vi "MathCad cmd v2.vi"(4 "Arr Refnum":refnum<vi>, 5 "MathCAD variables":T1, 6 "MathCAD cmds":T2, 7 "Str Refnum":refnum<vi>, 8 "error in":errorcluster, 9 "Clust Refnum":refnum<vi>, 10 "Num Refnum":refnum<vi>) -> (0 "first error out":errorcluster, 1 "errors":errorcluster[](array[cluster]))   [LabVIEW 2011, in "Design Server.lvlib"]
uses:
  Design Server.lvlib
  MathCAD cmd.ctl
  MathCAD results ref.ctl
panel:
  in  "Worksheet":path=path "C:/Users/design/Documents/Final Designs/AguaClaraDesignTool.xmcd"
  in  "Mathcad.IMathcadApplication":refnum<k7>
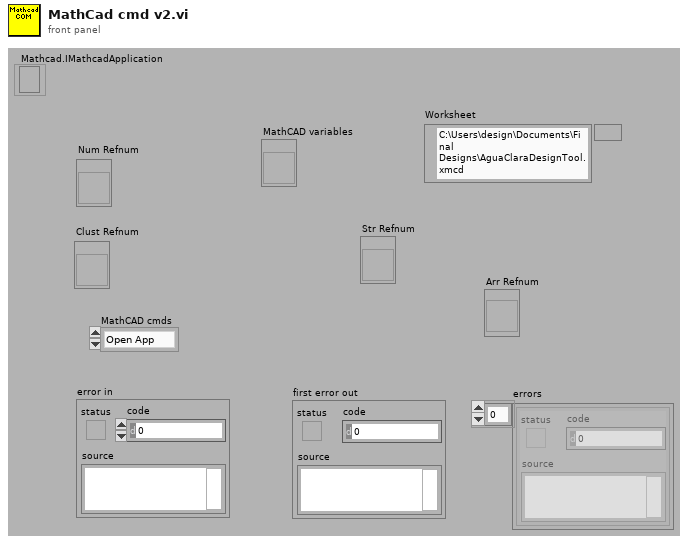
[diagram p1: front panel]
types:
  T1 = typedef "Design Server.lvlib/MathCAD results ref.ctl" = refnum<vi>
  T2 = typedef "Design Server.lvlib/MathCAD cmd.ctl" = enum16{"Open App", "Open Worksheet", "Close Worksheet", "Load Variable Ref", "Send Number", "Send Cluster", "Send Array", "Send String", "Calculate", "Get MathCAD data", "Close MathCAD"}
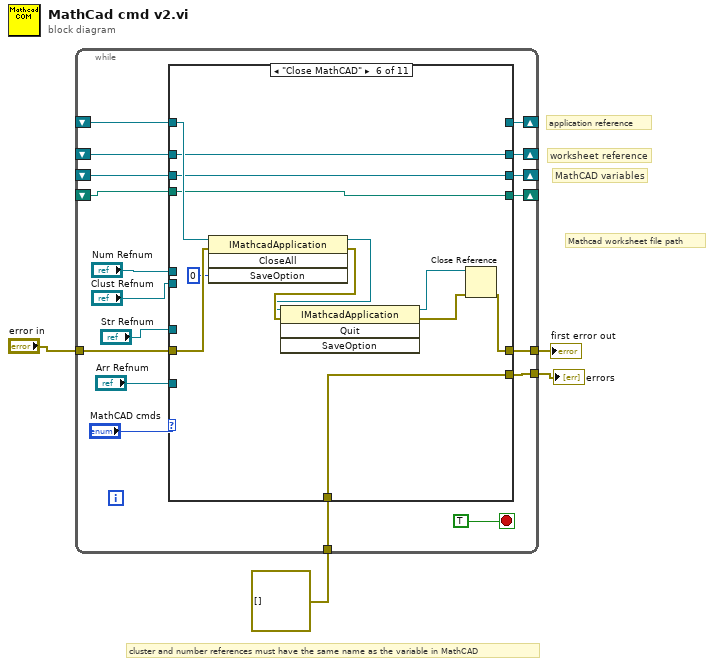
[diagram p0: block diagram]
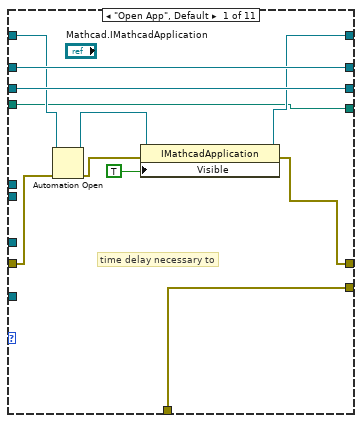
[diagram p2: hidden frame]
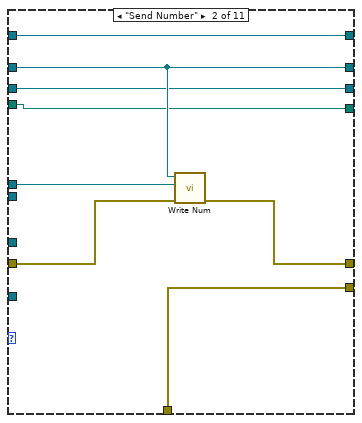
[diagram p3: hidden frame]
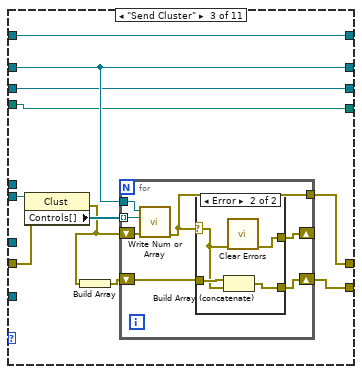
[diagram p4: hidden frame]
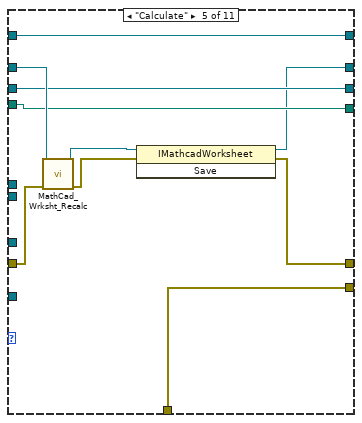
[diagram p7: hidden frame]
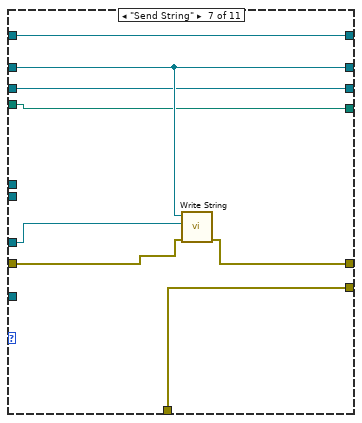
[diagram p8: hidden frame]
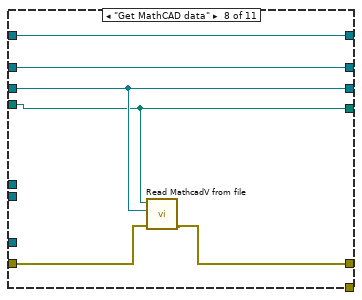
[diagram p9: hidden frame]
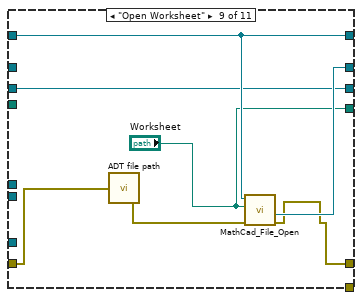
[diagram p10: hidden frame]
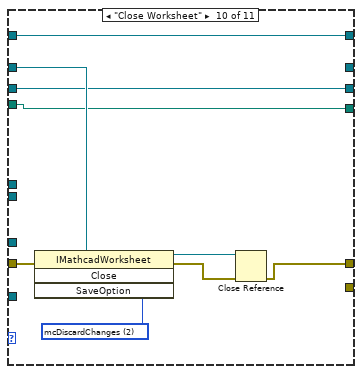
[diagram p11: hidden frame]
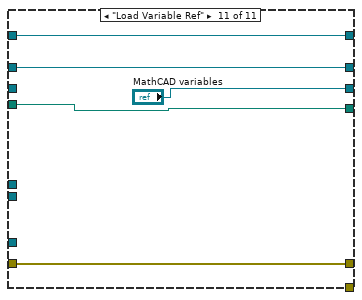
[diagram p12: hidden frame]
diagram:
  # "Mathcad worksheet file path"
  # "MathCAD variables"
  # "application reference"
  # "worksheet reference"
  # "cluster and number references must have the same name as the variable in MathCAD"
  n1 = while {
    shift-right: [w18] -> _
    shift-left: _ -> [w16]
    shift-right: [w17] -> _
    shift-left: _ -> [w15]
    tunnel: "error in" -> [w19]
    tunnel: [w20] -> w3
    tunnel: [w10] -> w2
    tunnel: errorcluster[] [] -> [w9]
    shift-right: [w8] -> _
    shift-left: _ -> [w7]
    shift-right: [w6] -> _
    shift-left: _ -> [w5]
    stop <- TRUE stop-if-true
    n2 = case shown="\"Close MathCAD\"" "MathCAD cmds" {
      tunnel: [w26 w38 w49 w69 w72 w88 w99 w104 w109 w116 w125] -> w20
      tunnel: w19 -> [w25 w40 w47 w69 w79 w92 w100 w105 w112 w123 w125]
      tunnel: [w27 w41 w51 w71 w81 _ w101 w107 w114 w120 w126] -> w18
      tunnel: [w32 w39 w50 w70 w74 w91 w97 w106 w113 _ w127] -> w17
      tunnel: w16 -> [w30 w41 w51 w71 w81 w93 w101 w107 w114 w120 w126]
      tunnel: w15 -> [w32 w39 w50 w70 w80 w91 w97 w106 _ w121 w127]
      tunnel: "Num Refnum" -> [_ w37 _ _ _ _ _ _ _ _ _]
      tunnel: "Clust Refnum" -> [_ _ w48 _ _ _ _ _ _ _ _]
      tunnel: "Str Refnum" -> [_ _ _ _ _ _ w98 _ _ _ _]
      tunnel: "Arr Refnum" -> [_ _ _ _ _ _ _ _ _ _ _]
      tunnel: [w33 w36 w44 w68 w78 w90 w96 _ _ _ _] -> w10
      tunnel: w9 -> [w33 w36 _ w68 w78 w90 w96 _ _ _ _]
      tunnel: w7 -> [w31 w35 w43 w67 w77 w89 w95 w103 w110 w119 _]
      tunnel: [w31 w35 w43 w67 w77 w89 w95 w103 w110 w119 "MathCAD variables"] -> w8
      tunnel: [w23 w34 w42 w66 w76 w82 w94 w102 "Worksheet" w115 w124] -> w6
      tunnel: w5 -> [w23 w34 w42 w66 w76 w82 w94 w102 _ w115 w124]
      frame "Open App", Default {
        # "time delay necessary to"
        n3 = Automation Open(error in (no error)=w25, Automation Refnum=w30) -> (Automation Refnum=w29:refnum<k7>, error out=w28:errorcluster)  [unwired: 2 in]
        n4 = property class="IMathcadApplication"(reference=w29, error in=w28, "Visible"=TRUE) -> (reference out=w27:refnum<k7>, error out=w26:errorcluster)
      }
      frame "Send Number" {
        n5 = call "Write Num.vi"("error in (no error)"=w40, "Ctl Refnum"=w37, "Worksheet Reference"=w39) -> ("error out"=w38:errorcluster)  [unwired: 8 in]
      }
      frame "Send Cluster" {
        n6 = property class="Clust"(reference=w48, error in=w47) -> (error out=w46:errorcluster, "Controls[]"=w52:refnum<vi>[])  [unwired: 1 out]
        n7 = Build Array(w46) -> (w45:errorcluster[])
        n8 = for {
          tunnel: w52 -> [w55] mode=indexing
          tunnel: w50 -> [w54]
          tunnel: [w53] -> w49
          shift-right: [w57] -> _
          shift-left: w46 -> [w56]
          shift-right: [w58] -> w44
          shift-left: w45 -> [w59]
          n9 = call "Write Num or Array.vi"("error in (no error)"=w56, "Ctl Refnum"=w55, "Worksheet Reference"=w54) -> ("error out"=w53:errorcluster)  [unwired: 8 in]
          n10 = case shown="Error" w53 {
            selector: w53 -> [w60 w63]
            tunnel: w59 -> [w61 w65]
            tunnel: [w61 w64] -> w58
            tunnel: [w60 w62] -> w57
            frame No Error {
            }
            frame Error {
              n11 = Build Array (concatenate)(w65, w63) -> (w64:errorcluster[])
              n12 = call <vilib>:"Clear Errors.vi"("error in (no error)"=w63) -> ("error out"=w62:errorcluster)  [unwired: 6 in]
            }
          }
        }
      }
      frame "Send Array" {
      }
      frame "Calculate" {
        n13 = call "MathCad_Wrksht_Recalc.vi"("error in (no error)"=w79, "Worksheet Reference"=w80) -> ("error out"=w73:errorcluster, "Worksheet Reference"=w75:refnum<k7>)  [unwired: 8 in]
        n14 = invoke class="IMathcadWorksheet" method="Save"(reference=w75, error in=w73) -> (reference out=w74:refnum<k7>, error out=w72:errorcluster)  [unwired: 1 in, 1 out]
      }
      frame "Close MathCAD" {
        n15 = invoke class="IMathcadApplication" method="CloseAll"(reference=w93, error in=w92, "SaveOption"=0) -> (reference out=w86:refnum<k7>, error out=w87:errorcluster)  [unwired: 1 in, 2 out]
        n16 = invoke class="IMathcadApplication" method="Quit"(reference=w86, error in=w87) -> (reference out=w85:refnum<k7>, error out=w84:errorcluster)  [unwired: 2 in, 2 out]
        n17 = Close Reference(reference=w85, error in (no error)=w84) -> (error out=w88:errorcluster)
      }
      frame "Send String" {
        n18 = call "Write String.vi"("error in (no error)"=w100, "Ctl Refnum"=w98, "Worksheet Reference"=w97) -> ("error out"=w99:errorcluster)  [unwired: 8 in]
      }
      frame "Get MathCAD data" {
        n19 = call "Read MathcadV from file.vi"("error in (no error)"=w105, 10:w103, "Path"=w102) -> ("error out"=w104:errorcluster)  [unwired: 7 in, 1 out]
      }
      frame "Open Worksheet" {
        n20 = call "ADT file path.vi"("error in"=w112) -> ("error out"=w111:errorcluster)  [unwired: 1 out]
        n21 = call "MathCad_File_Open.vi"("error in (no error)"=w111, "Worksheet File"="Worksheet", "Mathcad.IMathcadApplication"=w114) -> ("error out (no error)"=w109:errorcluster, "Worksheet Reference"=w113:refnum<k7>)  [unwired: 5 in, 2 out]
      }
      frame "Close Worksheet" {
        w122 = 2 items=["mcSaveChanges", "mcPromptToSaveChanges", "mcDiscardChanges"] ("SaveOption")
        n22 = invoke class="IMathcadWorksheet" method="Close"(reference=w121, error in=w123, "SaveOption"=w122) -> (reference out=w118:refnum<k7>, error out=w117:errorcluster)  [unwired: 1 in, 2 out]
        n23 = Close Reference(reference=w118, error in (no error)=w117) -> (error out=w116:errorcluster)
      }
      frame "Load Variable Ref" {
      }
    }
  }
  "first error out" <- w3
  "errors" <- w2
